vi "Column Headers.vi"(8 "error in (no error)":errorcluster, 11 "TestStand Result Handler in":refnum<class "TestStand Result Handler.lvclass">) -> (0 "error out":errorcluster, 2 "Array":string[](array[string]), 3 "TestStand Result Handler out":refnum<class "TestStand Result Handler.lvclass">)   [LabVIEW 2020, in "Astemes_CSVReportPlugin.lvlib" / "TestStand Result Handler.lvclass"]
doc: "Template method for generating column headers. Use this to ensure column headers are matching any results added using additional results."
uses:
  TestStand Result Handler.lvclass
  Private/Columns.ctl
  19c64cdd-03c9-45ee-ba45-2cb337f8b74a.vi
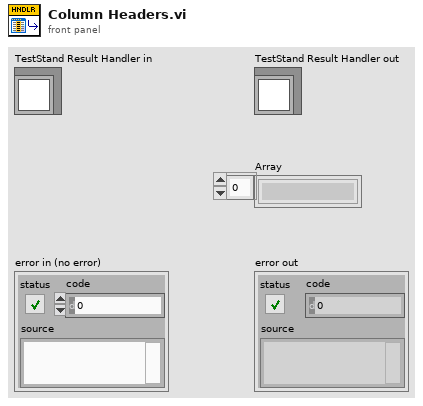
[diagram p1: front panel]
types:
  T1 = typedef "Astemes_CSVReportPlugin.lvlib/TestStand Result Handler.lvclass/Columns.ctl" = enum16{"StepName", "Result", "LowerLimit", "ComparisonTypeLow", "Measurement", "ComparisonTypeHigh", "UpperLimit", "ReportText", "StepType"}
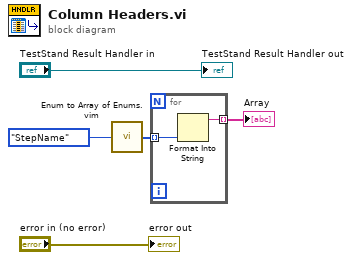
[diagram p0: block diagram]
diagram:
  n1 = call "Enum to Array of Enums.vim"("enum"=Columns."StepName" ("Column")) -> ("array of enums"=w1:T1[])
  n2 = for {
    tunnel: w1 -> [w7] mode=indexing
    tunnel: [w6] -> w3 mode=indexing
    n3 = Format Into String(w7) -> (resulting string=w6:string)  [unwired: 3 in, 1 out]
  }
  "Array" <- w3
  "error out" <- "error in (no error)"
  "TestStand Result Handler out" <- "TestStand Result Handler in"
